vi "create and send sql query expt editor scan start end SRS delays.vi"(8 "error in (no error)":errorcluster, 10 "Array":T1[](array[typedef]) {"Scan End" format="%#_6p"; "Scan Start" format="%#_6p"}, 11 "exptdeviceID":string) -> (0 "error out":errorcluster)   [LabVIEW 2020]
uses:
  Bella center GUIs/GUI_Bella_BTL/delay scan start and end.ctl
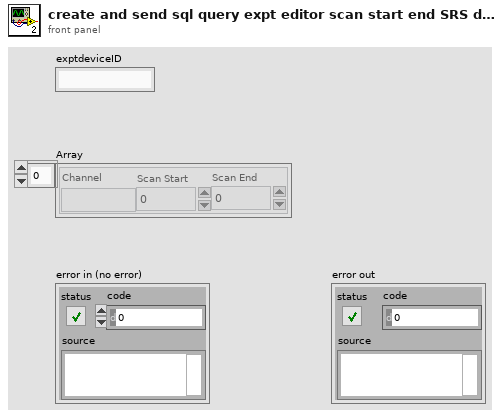
[diagram p1: front panel]
types:
  T1 = typedef "delay scan start and end.ctl" = cluster{"Channel":string, "Scan Start":dbl, "Scan End":dbl}
  T2 = typedef "mysql_authentication.ctl" = cluster{"User":string, "Password":string, "Database":string}
  T3 = cluster{"Port":u16, "IP Address":string, "Authentication":T2}
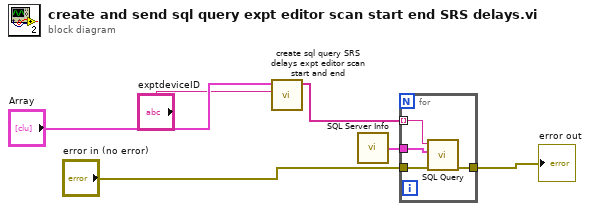
[diagram p0: block diagram]
diagram:
  n1 = call "create sql query SRS delays expt editor scan start and end.vi"("exptdeviceID"="exptdeviceID", "Expt editor SCS on"="Array") -> ("Array"=w6:string[])  [unwired: 9 in]
  n2 = call "SQL Server Info.vi"() -> ("SQL Server Info"=w3:T3)
  n3 = for {
    tunnel: w6 -> [w10] mode=indexing
    tunnel: w3 -> [w9]
    tunnel: "error in (no error)" -> [w8]
    tunnel: [w7] -> w5
    n4 = call "SQL Query.vi"("error in (no error)"=w8, "SQL Server Info"=w9, "Query"=w10) -> ("error out"=w7:errorcluster)  [unwired: 7 in, 1 out]
  }
  "error out" <- w5
